vi "sub_vi_set_linear_parameters.vi"(5 "intercept":dbl, 7 "slope":dbl, 8 "error in (no error)":errorcluster, 10 "gain":i32, 11 "VISA resource name in":refnum<visa-resource-name>) -> (0 "error out":errorcluster, 1 "Writing to EEPROM":bool, 2 "read buffer":string, 3 "VISA resource name out":refnum<visa-resource-name>)   [LabVIEW 2016]
panel:
  out "command string":string
  out "concatenated string":string
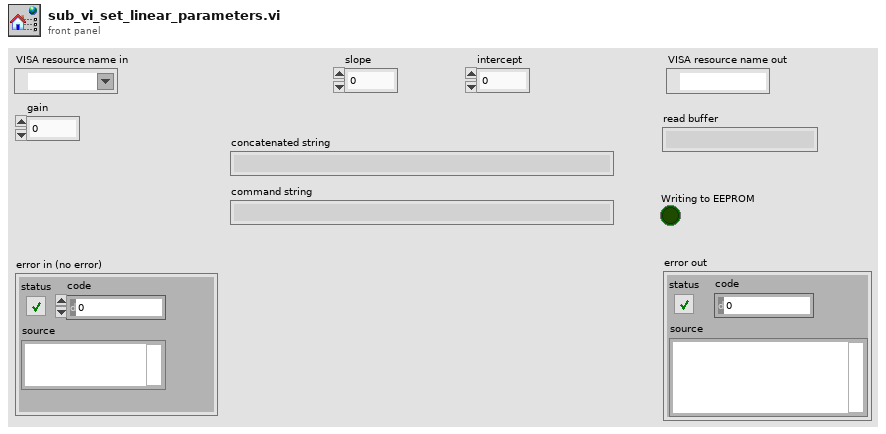
[diagram p1: front panel]
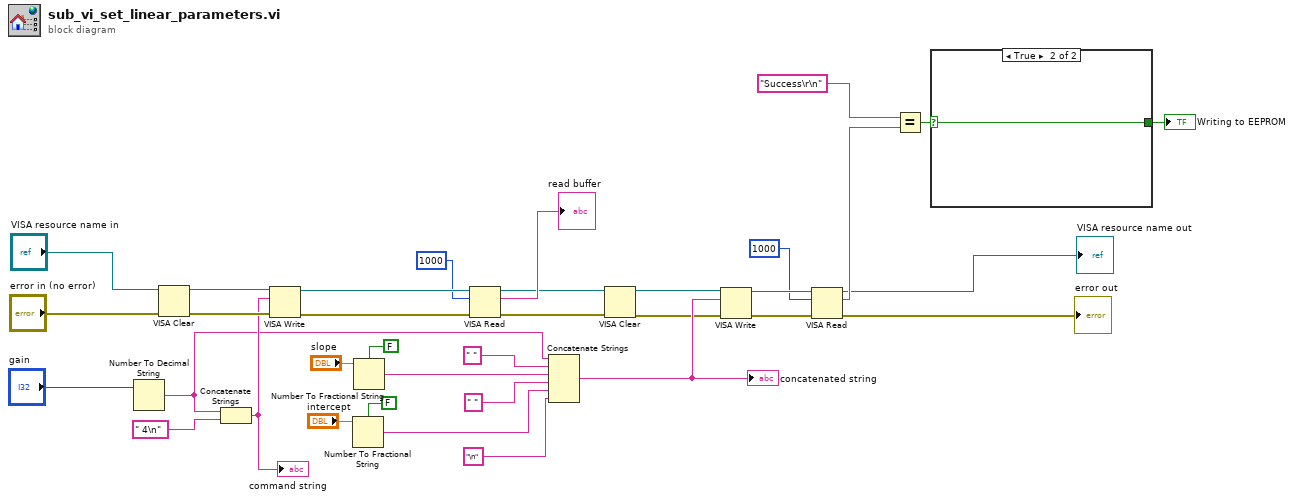
[diagram p0: block diagram]
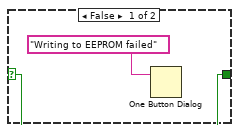
[diagram p2: hidden frame]
diagram:
  n1 = Number To Decimal String(number="gain") -> (decimal integer string=w8:string)  [unwired: 1 in]
  n2 = VISA Clear(VISA resource name="VISA resource name in", error in (no error)="error in (no error)") -> (VISA resource name out=w35:refnum<visa-resource-name>, error out=w34:errorcluster)
  n3 = Concatenate Strings(w8, " 4\n" ("string")) -> (w29:string)
  "command string" <- w29
  n4 = VISA Write(VISA resource name=w35, write buffer=w29, error in (no error)=w34) -> (VISA resource name out=w14:refnum<visa-resource-name>, error out=w13:errorcluster)  [unwired: 1 out]
  n5 = Number To Fractional String(use system decimal point (T)=FALSE, number="intercept") -> (F-format string=w24:string)  [unwired: 2 in]
  n6 = Number To Fractional String(use system decimal point (T)=FALSE, number="slope") -> (F-format string=w26:string)  [unwired: 2 in]
  n7 = VISA Read(VISA resource name=w14, byte count=u32 1000, error in (no error)=w13) -> (VISA resource name out=w7:refnum<visa-resource-name>, read buffer=→"read buffer":string, error out=w4:errorcluster)  [unwired: 1 out]
  n8 = Concatenate Strings(w8, " " ("string"), w26, " " ("string"), w24, "\n" ("string")) -> (w22:string)
  "concatenated string" <- w22
  n9 = VISA Clear(VISA resource name=w7, error in (no error)=w4) -> (VISA resource name out=w6:refnum<visa-resource-name>, error out=w5:errorcluster)
  n10 = VISA Write(VISA resource name=w6, write buffer=w22, error in (no error)=w5) -> (VISA resource name out=w33:refnum<visa-resource-name>, error out=w32:errorcluster)  [unwired: 1 out]
  n11 = VISA Read(VISA resource name=w33, byte count=u32 1000, error in (no error)=w32) -> (VISA resource name out=→"VISA resource name out":refnum<visa-resource-name>, read buffer=w19:string, error out=→"error out":errorcluster)  [unwired: 1 out]
  n12 = Equal?(x="Success\r\n" ("y"), y=w19) -> (x = y?=w21:bool)
  n13 = case shown="True" w21 {
    selector: w21 -> [w36 w38]
    tunnel: [w36 w38] -> w1
    frame False {
      n14 = One Button Dialog(message="Writing to EEPROM failed") -> ()  [unwired: 1 in, 1 out]
    }
    frame True {
    }
  }
  "Writing to EEPROM" <- w1
